vi "MedianFilter.vi"(2 "Reverse":bool, 3 "Invert?":bool=TRUE, 4 "Replace value":u8, 5 "data in":u8[][][](array[numeric]), 6 "window size":i32=10, 7 "threshold":i32) -> (1 "data out":u8[][][](array[numeric]))   [LabVIEW 2022 SP3]
uses:
  <vilib>/Analysis/NI_AALBase.lvlib
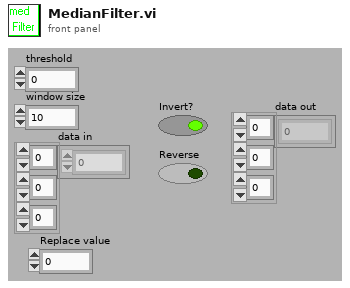
[diagram p1: front panel]
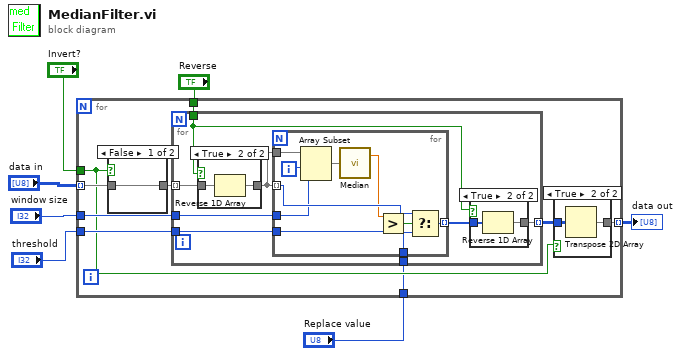
[diagram p0: block diagram]
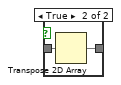
[diagram p2: hidden frame]
diagram:
  n1 = for {
    tunnel: "data in" -> [w15] mode=indexing
    tunnel: [w13] -> w4 mode=indexing
    tunnel: "window size" -> [w12]
    tunnel: "threshold" -> [w11]
    tunnel: "Invert?" -> [w10]
    tunnel: "Reverse" -> [w9]
    tunnel: "Replace value" -> [w8]
    n2 = case shown="False" w10 {
      tunnel: w15 -> [w17 w19]
      tunnel: [w17 w18] -> w14
      frame False {
      }
      frame True {
        n3 = Transpose 2D Array(2D array=w19) -> (transposed array=w18:u8[][])
      }
    }
    n4 = for {
      tunnel: w14 -> [w30] mode=indexing
      tunnel: [w25] -> w16 mode=indexing
      tunnel: w12 -> [w28]
      tunnel: w11 -> [w27]
      tunnel: w9 -> [w24]
      tunnel: w8 -> [w23]
      n5 = case shown="True" w24 {
        tunnel: w30 -> [w31 w33]
        tunnel: [w31 w32] -> w26
        frame False {
        }
        frame True {
          n6 = Reverse 1D Array(array=w33) -> (reversed array=w32:u8[])
        }
      }
      n7 = for {
        tunnel: w26 -> [w43] mode=indexing
        tunnel: w26 -> [w46]
        tunnel: [w41] -> w29 mode=indexing
        tunnel: w28 -> [w39]
        tunnel: w27 -> [w38]
        tunnel: w23 -> [w37]
        i -> [w45]
        n8 = Array Subset(array=w46, index=w45, length=w39) -> (w42:u8[])
        n9 = call <vilib>:"Median.vi"("X"=w42) -> ("median"=w40:dbl)  [unwired: 1 out]
        n10 = Greater?(x=w40, y=w38) -> (0:w44:bool)
        n11 = Select(t=w43, s=w44, f=w37) -> (s? t:f=w41:u8)
      }
      n12 = case shown="True" w24 {
        tunnel: w29 -> [w34 w36]
        tunnel: [w34 w35] -> w25
        frame False {
        }
        frame True {
          n13 = Reverse 1D Array(array=w36) -> (reversed array=w35:u8[])
        }
      }
    }
    n14 = case shown="True" w10 {
      tunnel: w16 -> [w20 w22]
      tunnel: [w20 w21] -> w13
      frame False {
      }
      frame True {
        n15 = Transpose 2D Array(2D array=w22) -> (transposed array=w21:u8[][])
      }
    }
  }
  "data out" <- w4
